vi "TEST - Flush Msg Queue.vi"(8 "error in (no error)":errorcluster) -> (0 "error out":errorcluster, 2 "pass":bool)   [LabVIEW 2009]
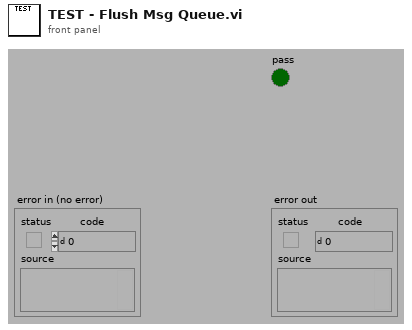
[diagram p1: front panel]
types:
  T1 = typedef "Msg Queue RefNum.ctl" = refnum<k1>
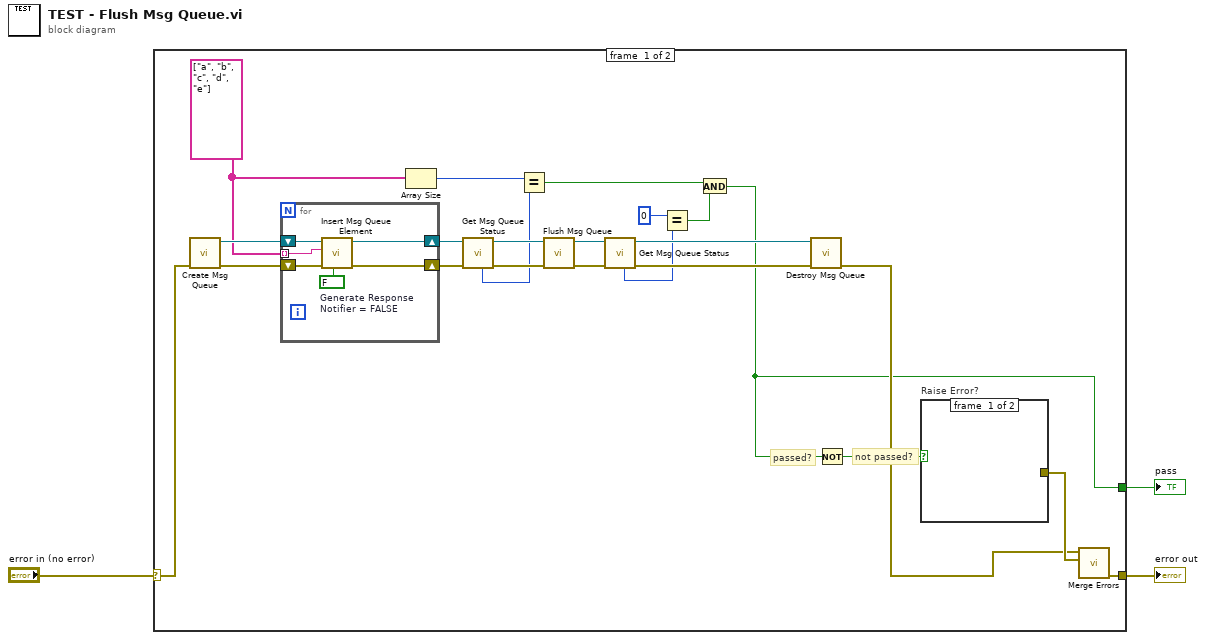
[diagram p0: block diagram]
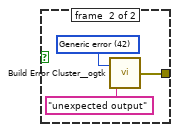
[diagram p2: hidden frame]
diagram:
  n1 = case shown="No Error" "error in (no error)" {
    selector: "error in (no error)" -> [w20 w36]
    tunnel: [w6 _] -> w3
    tunnel: [w26 w36] -> w1
    frame #0 {
      w16 = string[] ["a", "b", "c", "d", "e"]
      # "not passed?"
      # "passed?"
      n2 = call "Create Msg Queue.vi"("error in (no error)"=w20) -> ("error out"=w23:errorcluster, "msg queue"=w19:T1)  [unwired: 4 in, 1 out]
      n3 = for {
        tunnel: w16 -> [w32] mode=indexing
        shift-right: [w30] -> w18
        shift-left: w19 -> [w31]
        shift-right: [w28] -> w17
        shift-left: w23 -> [w29]
        w27 = FALSE  # Generate Response Notifier = FALSE
        n4 = call "Insert Msg Queue Element.vi"("Generate Response Notifier (F)"=w27, "error in (no error)"=w29, "message"=w32, "msg queue"=w31) -> ("error out"=w28:errorcluster, "msg queue out"=w30:T1)  [unwired: 2 in, 2 out]
      }
      n5 = Array Size(array=w16) -> (size(s)=w15:i32)
      n6 = call "Get Msg Queue Status.vi"("error in (no error)"=w17, "msg queue"=w18) -> ("error out"=w13:errorcluster, "msg queue out"=w14:T1, "# elements in queue"=w5:i32)  [unwired: 2 in, 5 out]
      n7 = Equal?(x=w15, y=w5) -> (x = y?=w8:bool)
      n8 = call "Flush Msg Queue.vi"("error in (no error)"=w13, "msg queue"=w14) -> ("error out"=w11:errorcluster, "msg queue out"=w12:T1)  [unwired: 3 in, 1 out]
      n9 = call "Get Msg Queue Status.vi"("error in (no error)"=w11, "msg queue"=w12) -> ("error out"=w22:errorcluster, "msg queue out"=w7:T1, "# elements in queue"=w4:i32)  [unwired: 2 in, 5 out]
      n10 = Equal?(x=0, y=w4) -> (x = y?=w9:bool)
      n11 = And(x=w8, y=w9) -> (x .and. y?=w6:bool)
      n12 = call "Destroy Msg Queue.vi"("error in (no error)"=w22, "msg queue"=w7) -> ("error out"=w21:errorcluster)  [unwired: 3 in, 2 out]
      n13 = Not(x=w6) -> (.not. x?=w24:bool)
      n14 = case "Raise Error?" shown="True" w24 {
        tunnel: [_ w33] -> w25
        frame #0 {
        }
        frame #1 {
          w34 = 42 items=["No error", "Argument error", "Memory is full", "Out of zone", "End of file", "File already open", "Generic file I/O error", "File not found", "File permission error", "Disk is full", "Duplicate path", "Too many files open", "System feature not enabled", "Resource file not found", "Cannot add resource", "Resource not found", "Image not found", "Image memory error", "Pen does not exist", "Config type invalid", "Config token not found", "Config parse error", "Config memory error", "Bad external code format", "Bad external code offset", "External code not present", "Null window", "Destroy window error", "Null menu", "Print aborted", "Bad print record", "Print driver error", "Windows error during printing", "Memory error during printing", "Print dialog error", "Generic print error", "Invalid device refnum", "Device not found", "Device parameter error", "Device unit error", "Cannot open device", "Device call aborted", "Generic error", "Cancelled by user", "Object ID too low", "Object ID too high", "Object not in heap", "Unknown heap", "Unknown object (invalid DefProc)", "Unknown object (DefProc not in table)", "Message out of range", "Invalid (null) method", "Unknown message", "Manager call not supported", "Bad address", "Network operation in progress", "Network operation timed out", "Connection is busy", "Network attribute not supported", "Network error", "Address in use", "System out of memory", "Connection aborted", "Connection refused", "Not connected", "Already connected", "Connection closed", "Initialization error (interapplication manager)", "Bad occurrence", "Wait on unbound occurrence handler", "Occurrence queue overflow", "Datalog type conflict", "Unused", "Unrecognized type (interapplication manager)", "Memory corrupt", "Failed to make temporary DLL", "Old CIN version", "Drag socket not found", "Failed to load drop-object", "Failed to register OLE object", "Failed to release OLE object", "Format specifier type mismatch", "Unknown format specifier", "Too few format specifiers", "Too many format specifiers", "Scan failed", "Newer CIN version", "Error converting to variant", "Runtime menu error", "Password tampered", "Variant attribute not found", "Incompatible variant data type", "Event data is not available", "Event Store is not present", "Occurrence is not found", "Event Queue is not created", "Event info is not available", "Refnum passed is NULL", "Error retrieving Class GUID", "Error retrieving CoClass GUID", "Error retrieving TypeLib GUID.", "Bad built application magic bytes.", "Specific driver is different from the specific driver associated with the Logical Name.", "There is no session opened to the class driver.", "Max Error", "MAX - Error with config objects", "MAX - Error loading configuration", "MAX - Group not supported"]
          n15 = call <userlib>:"Build Error Cluster__ogtk.vi"("String to Prepend to source (\"\")"="unexpected output" ("String to Prepend to source (\"\")"), "code"=w34) -> ("error out"=w33:errorcluster)
        }
      }
      n16 = call <vilib>:"Merge Errors.vi"("error in 2 (no error)"=w25, "error in 1 (no error)"=w21) -> ("error out"=w26:errorcluster)  [unwired: 5 in]
    }
    frame #1 {
    }
  }
  "pass" <- w3
  "error out" <- w1
